vi "File_OpenWfms.vi"(8 "error in (no error)":errorcluster, 11 "File in":refnum<class "File.lvclass">) -> (0 "error out":errorcluster, 3 "File out":refnum<class "File.lvclass">)   [LabVIEW 2023, in "File.lvclass"]
doc: "Top level VI that triggers waveform channels to get the waveform reference during compilation for use in the VeriStand Engine."
uses:
  File.lvclass
  File.lvclass/File.ctl
  Group/Group.lvclass
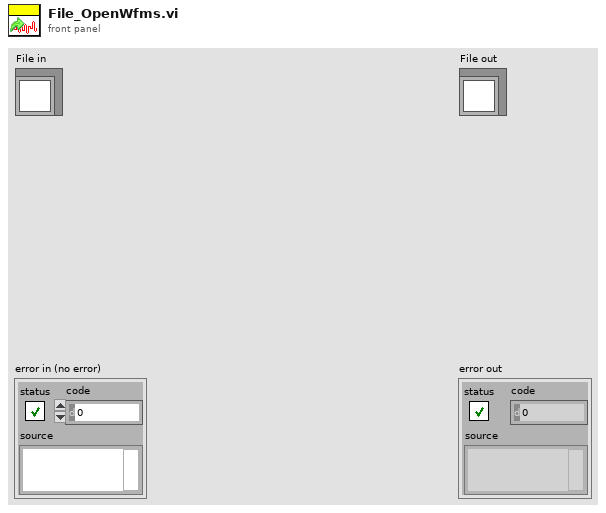
[diagram p1: front panel]
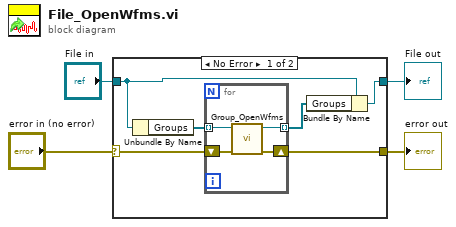
[diagram p0: block diagram]
diagram:
  n1 = case shown="No Error" "error in (no error)" {
    selector: "error in (no error)" -> [w6 w16]
    tunnel: [w5 w16] -> w3
    tunnel: [w9 w15] -> w1
    tunnel: "File in" -> [w10 w15]
    frame No Error {
      n2 = Unbundle By Name(w10) -> ("Groups"=w8:refnum<class "Group.lvclass">[])
      n3 = for {
        tunnel: w8 -> [w14] mode=indexing
        tunnel: [w13] -> w7 mode=indexing
        shift-right: [w12] -> w5
        shift-left: w6 -> [w11]
        n4 = call-dynamic "Group_OpenWfms.vi"("error in (no error)"=w11, "Group in"=w14) -> ("error out"=w12:errorcluster, "Group out"=w13:refnum<class "Group.lvclass">)  [unwired: 8 in]
      }
      n5 = Bundle By Name(cluster=w10, "Groups"=w7) -> (w9:refnum<class "File.lvclass">)
    }
    frame Error {
    }
  }
  "error out" <- w3
  "File out" <- w1
